vi "U16转换为float.vi"(6 "第几组数据":i32, 7 "选择?":bool[](array[boolean]), 8 "低16位_2":u16, 9 "高16位_2":u16, 10 "低16位_1":u16, 11 "高16位_1":u16) -> (0 "反馈值2":dbl, 1 "反馈值1":dbl, 2 "反馈值字符_2":string, 3 "反馈值字符_1":string)   [LabVIEW 2010]
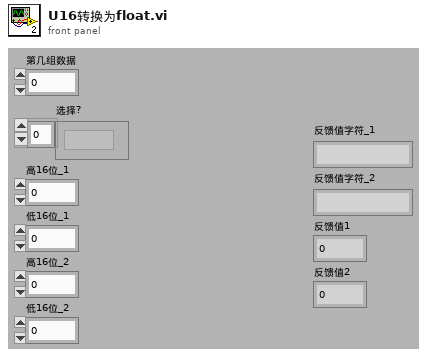
[diagram p1: front panel]
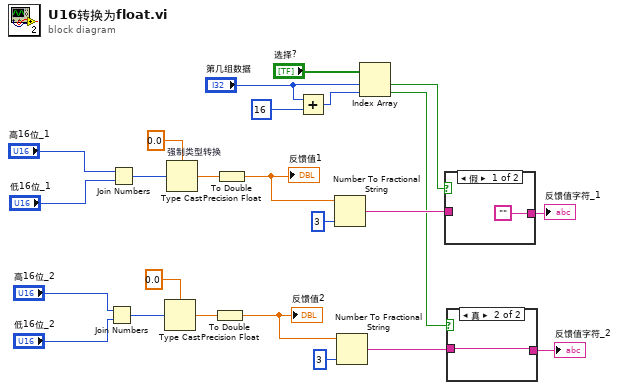
[diagram p0: block diagram]
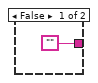
[diagram p2: hidden frame]
diagram:
  n1 = Join Numbers(hi="高16位_2", lo="低16位_2") -> ((hi.lo)=w18:u32)
  n2 = Join Numbers(hi="高16位_1", lo="低16位_1") -> ((hi.lo)=w21:u32)
  n3 = Type Cast(type=sgl 0.0, x=w18) -> (*(type *) &x=w19:sgl)
  n4 = Type Cast "强制类型转换"(type=sgl 0.0, x=w21) -> (*(type *) &x=w20:sgl)
  n5 = To Double Precision Float(number=w19) -> (double precision float=w7:dbl)
  "反馈值2" <- w7
  n6 = To Double Precision Float(number=w20) -> (double precision float=w13:dbl)
  "反馈值1" <- w13
  n7 = Add(x="第几组数据", y=16) -> (x+y=w9:i32)
  n8 = Number To Fractional String(number=w13, precision (6)=i16 3 ("精度(6)")) -> (F-format string=w5:string)  [unwired: 2 in]
  n9 = Number To Fractional String(number=w7, precision (6)=i16 3 ("精度(6)")) -> (F-format string=w1:string)  [unwired: 2 in]
  n10 = Index Array(array="选择?", index #1="第几组数据", index #2=w9) -> (element #1=w3:bool, element #2=w2:bool)
  n11 = case shown="假" w3 {
    tunnel: ["" w26] -> w6
    tunnel: w5 -> [_ w26]
    frame False {
    }
    frame True {
    }
  }
  "反馈值字符_1" <- w6
  n12 = case shown="真" w2 {
    tunnel: ["" w28] -> w4
    tunnel: w1 -> [_ w28]
    frame False {
    }
    frame True {
    }
  }
  "反馈值字符_2" <- w4
